vi "sub_alarm.vi"(7 "alarm":T1(ring)) -> ()   [LabVIEW 2019]
uses:
  Devices/NI Board/cDAQ-9476 DO/cnt_Relay.ctl
  Durability/common/Global 1.vi
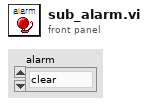
[diagram p1: front panel]
types:
  T1 = enum16{"clear", "Red", "Yellow", "Beep", "Beep onoff"}
  T2 = typedef "cnt_Relay.ctl" = enum32{"R_Load", "R_out1", "R_out2", "R_out3", "R_out4", "R_out5", "R_out6", "R8", "R9", "R10", "R11", "R12", "R13", "R14", "R15", "R16", "R_in1", "R_in2", "R_in3", "R_in4", "R_in5", "R_in6", "R23", "R24", "R25", "R26", "R27", "R_red", "R_yellow", "R_green", "R_buz", "R_purple"}
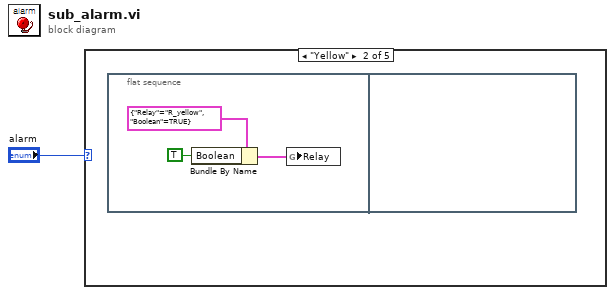
[diagram p0: block diagram]
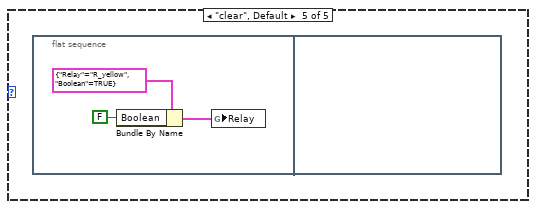
[diagram p5: hidden frame]
diagram:
  n1 = case shown="\"Yellow\"" "alarm" {
    frame "Red" {
    }
    frame "Yellow" {
      n2 = flat-sequence {
        frame #0 {
          n3 = Bundle By Name(cluster=cluster{"Relay":T2, "Boolean":bool} {"Relay"=enum."R_yellow", "Boolean"=TRUE} ("Relay"), "Boolean"=TRUE) -> (w2:cluster{"Relay":T2, "Boolean":bool})
          n4 = global write "Global 1.vi" "Relay"(w2) -> ()
        }
        frame #1 {
        }
      }
    }
    frame "Beep" {
    }
    frame "Beep onoff" {
    }
    frame "clear", Default {
      n5 = flat-sequence {
        frame #0 {
          n6 = Bundle By Name(cluster=cluster{"Relay":T2, "Boolean":bool} {"Relay"=enum."R_yellow", "Boolean"=TRUE} ("Relay"), "Boolean"=FALSE) -> (w5:cluster{"Relay":T2, "Boolean":bool})
          n7 = global write "Global 1.vi" "Relay"(w5) -> ()
        }
        frame #1 {
        }
      }
    }
  }
